vi "Disable VIO.vi"(0 "instrument handle":refnum<k15>, 5 "Bus Number":i32, 11 "error in":errorcluster) -> (4 "instrument handle out":refnum<k15>, 15 "error out":errorcluster)   [LabVIEW 2018, in "MIPI RFFE API.lvlib"]
uses:
  MIPI RFFE API.lvlib
  <instrlib>/niDigital/niDigital.llb/niDigital Selected Function.ctl
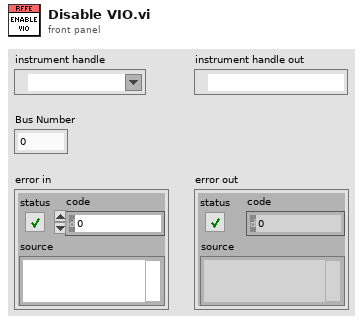
[diagram p1: front panel]
types:
  T1 = typedef "niDigital Selected Function.ctl" = i32
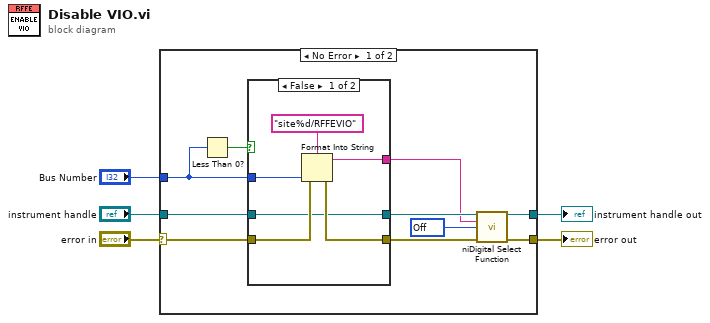
[diagram p0: block diagram]
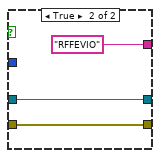
[diagram p2: hidden frame]
diagram:
  n1 = case shown="No Error" "error in" {
    selector: "error in" -> [w14 w26]
    tunnel: "instrument handle" -> [w11 w25]
    tunnel: [w8 w25] -> w4
    tunnel: [w10 w26] -> w2
    tunnel: "Bus Number" -> [w13 _]
    frame No Error {
      w6 = T1 1102 items=["Digital"=1100, "PPMU"=1101, "Off"=1102, "Disconnect"=1103] ("function")
      n2 = Less Than 0?(x=w13) -> (x < 0?=w15:bool)
      n3 = case shown="False" w15 {
        tunnel: w14 -> [w18 w23]
        tunnel: [w19 "RFFEVIO" ("channel list")] -> w7
        tunnel: w13 -> [w20 _]
        tunnel: [w17 w23] -> w12
        tunnel: w11 -> [w16 w22]
        tunnel: [w16 w22] -> w9
        frame False {
          n4 = Format Into String(format string="site%d/RFFEVIO" ("channel list"), error in=w18, w20) -> (resulting string=w19:string, error out=w17:errorcluster)  [unwired: 1 in]
        }
        frame True {
        }
      }
      n5 = call <instrlib>:"niDigital Select Function.vi"("instrument handle"=w9, "channel list"=w7, "function"=w6, "error in"=w12) -> ("instrument handle out"=w8:refnum<k15>, "error out"=w10:errorcluster)  [unwired: 10 in]
    }
    frame Error {
    }
  }
  "instrument handle out" <- w4
  "error out" <- w2
